vi "LHF.DB.Mongo.Collection.InsertVariant.vi"(6 "Extract ObjectID? (T)":bool=TRUE, 7 "ObjectID":string, 8 "error in (no error)":errorcluster, 9 "JSON Document":variant, 10 "Collection":string, 11 "LHF.DB.Mongo":refnum<class "LHF.DB.Mongo.lvclass">) -> (0 "error out":errorcluster, 2 "Inserted Document":string, 3 "LHF.DB.Mongo out":refnum<class "LHF.DB.Mongo.lvclass">, 5 "ObjectID out":string)   [LabVIEW 2013, in "LHF.DB.Mongo.lvclass"]
uses:
  LHF.DB.Mongo.lvclass
  C:/Users/schim/Desktop/Projetos/LabVIEW-MongoDB/src/Driver/MongoDB.Bson.dll
  Driver/MongoDB.Bson.dll
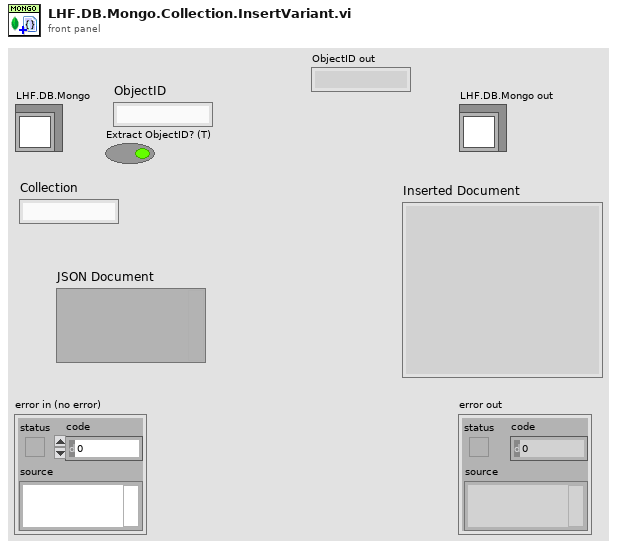
[diagram p1: front panel]
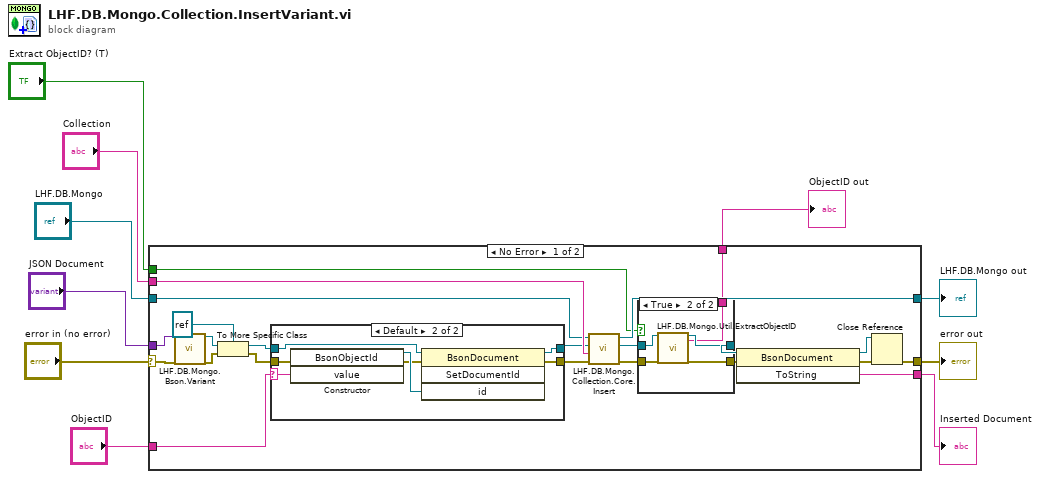
[diagram p0: block diagram]
diagram:
  n1 = case shown="No Error" "error in (no error)" {
    selector: "error in (no error)" -> [w31 w51]
    tunnel: [w28 w51] -> w9
    tunnel: [w32 w50] -> w7
    tunnel: "LHF.DB.Mongo" -> [w16 w50]
    tunnel: "JSON Document" -> [w23 _]
    tunnel: "Collection" -> [w33 _]
    tunnel: [w24 _] -> w4
    tunnel: "ObjectID" -> [w26 _]
    tunnel: "Extract ObjectID? (T)" -> [w18 _]
    tunnel: [w17 _] -> w1
    frame No Error {
      n2 = call "LHF.DB.Mongo.Bson.Variant.vi"("Variant"=w23, "error IO"=w31) -> ("BsonValue"=w27:refnum<k24>, "error IO 2"=w12:errorcluster)  [unwired: 16 in]
      n3 = To More Specific Class(target class=refnum<k24> refnum ("BsonDocument"), reference=w27, error in=w12) -> (specific class reference=w14:refnum<k24>, error out=w11:errorcluster)
      n4 = case shown="Default" w26 {
        selector: w26 -> [_ w46]
        tunnel: w14 -> [w42 w49]
        tunnel: [w42 w48] -> w15
        tunnel: w11 -> [w41 w45]
        tunnel: [w41 w43] -> w25
        frame "" {
        }
        frame Default {
          n5 = constructor class="BsonObjectId"(error in=w45, "value"=w46) -> (reference out=w47:refnum<k24>, error out=w44:errorcluster)  [unwired: 2 in, 2 out]
          n6 = invoke class="BsonDocument" method="SetDocumentId"(reference=w49, error in=w44, "id"=w47) -> (reference out=w48:refnum<k24>, error out=w43:errorcluster)  [unwired: 1 in, 2 out]
        }
      }
      n7 = call "LHF.DB.Mongo.Collection.Core.Insert.vi"("error in (no error)"=w25, "collectionName"=w33, "BsonDocument"=w15, "LHF.DB.Mongo in"=w16) -> ("error out"=w20:errorcluster, "BsonDocument out"=w22:refnum<k24>, "LHF.DB.Mongo out"=w32:refnum<class "LHF.DB.Mongo.lvclass">)  [unwired: 5 in]
      n8 = case shown="True" w18 {
        tunnel: w22 -> [w34 w40]
        tunnel: [w34 w39] -> w21
        tunnel: w20 -> [w35 w38]
        tunnel: [w35 w37] -> w19
        tunnel: [_ w36] -> w17
        frame False {
        }
        frame True {
          n9 = call "LHF.DB.Mongo.Util.ExtractObjectID.vi"("BsonDocument Refnum in"=w40, "error in (no error)"=w38) -> ("BsonDocument Refnum out"=w39:refnum<k24>, "ObjectID"=w36:string, "error out"=w37:errorcluster)  [unwired: 15 in]
        }
      }
      n10 = invoke class="BsonDocument" method="ToString"(reference=w21, error in=w19) -> (reference out=w30:refnum<k24>, error out=w29:errorcluster, "ToString"=w24:string)  [unwired: 1 in]
      n11 = Close Reference(reference=w30, error in (no error)=w29) -> (error out=w28:errorcluster)
    }
    frame Error {
    }
  }
  "error out" <- w9
  "LHF.DB.Mongo out" <- w7
  "Inserted Document" <- w4
  "ObjectID out" <- w1
